vi "壓縮機.vi"() -> ()   [LabVIEW 2022 SP3]
panel:
  out "Numeric 4":dbl
  out "Numeric 3":dbl
  out "Numeric 2":dbl
  out "開度 2":dbl
  out "開度":dbl
  in  "Slide":dbl(slide) min=0.0 max=192.0 step=12.0 scale=0.0..192.0
  out "Numeric":dbl
  in  "OK Button":bool
  # "壓縮機"
  # "比例閥-1"
  # "比例閥-2"
  # "%"
  # "%"
  # "HZ"
  # "流量計-1"
  # "流量計-2"
  # "流量計-3"
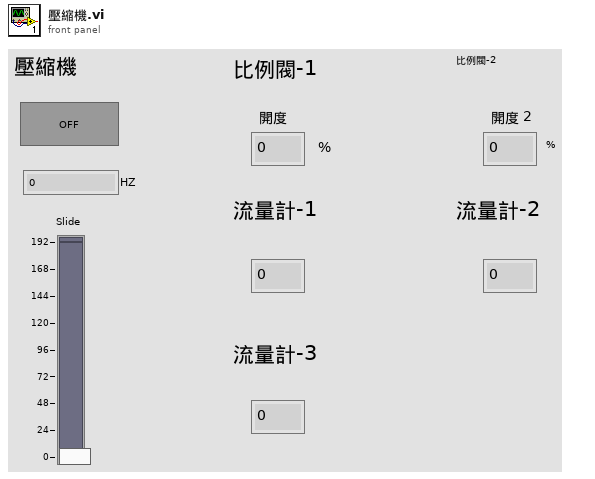
[diagram p1: front panel]
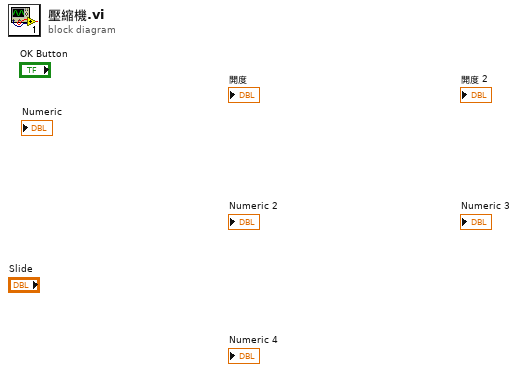
[diagram p0: block diagram]
diagram:
